vi "Resistivity_Calculation.vi"(3 "Reading 1 (V)":dbl, 4 "Constant":dbl, 5 "Thickness (nm)":dbl, 6 "Reading 2 (A)":dbl) -> (0 "Resivtivity (Ohm*cm)":dbl, 1 "Current":dbl, 2 "Voltage":dbl)   [LabVIEW 2010]
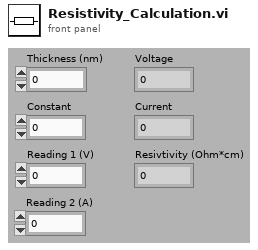
[diagram p1: front panel]
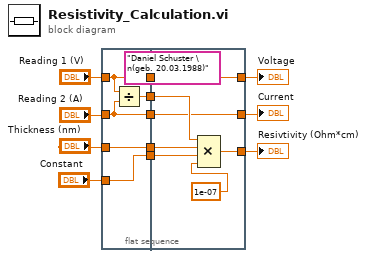
[diagram p0: block diagram]
diagram:
  (unwired) "Daniel Schuster \n(geb. 20.03.1988)"
  n1 = flat-sequence {
    tunnel: "Thickness (nm)" -> [w17]
    tunnel: [w17] -> w11
    tunnel: "Reading 1 (V)" -> [w14]
    tunnel: "Reading 2 (A)" -> [w13]
    tunnel: [w16] -> w8
    tunnel: [w15] -> w7
    tunnel: "Constant" -> [w15]
    tunnel: [w14] -> w4
    tunnel: [w13] -> w3
    tunnel: w11 -> [w24]
    tunnel: w8 -> [w23]
    tunnel: w7 -> [w21]
    tunnel: [w20] -> w5
    tunnel: [w19] -> w2
    tunnel: w4 -> [w19]
    tunnel: [w18] -> w1
    tunnel: w3 -> [w18]
    frame #0 {
      n2 = Divide(x=w14, y=w13) -> (x/y=w16:dbl)
    }
    frame #1 {
      n3 = Compound Arithmetic op=MULTIPLY(w23, w24, w21, 1e-07) -> (w20:dbl)
    }
  }
  "Resivtivity (Ohm*cm)" <- w5
  "Voltage" <- w2
  "Current" <- w1
